vi "Transcriptor LabVIEW to C code Engine 2.vi"(7 "VI path":path, 8 "Error In":errorcluster, 11 "Diagram in":refnum<vi>) -> (0 "Error Out":errorcluster, 1 "output cluster":T1, 2 "transcripted code":string, 3 "Diagram out":refnum<vi>, 5 "VI ref.":refnum<vi>)   [LabVIEW 2014]
uses:
  types/LabVIEW Universal Transcriptor Cluster.ctl
  types/LabVIEW Universal Transcriptor C code Composer Input Cluster.ctl
panel:
  out "FiringOrder":string[](array[string])
  # "0. create definitions (ClusterConstant)\n1. get all wires and create their declarations\n2. if wires are connected to control or constant assign value to them\n3. translate elements of diagram by firing order\n4. assign values to outputs"
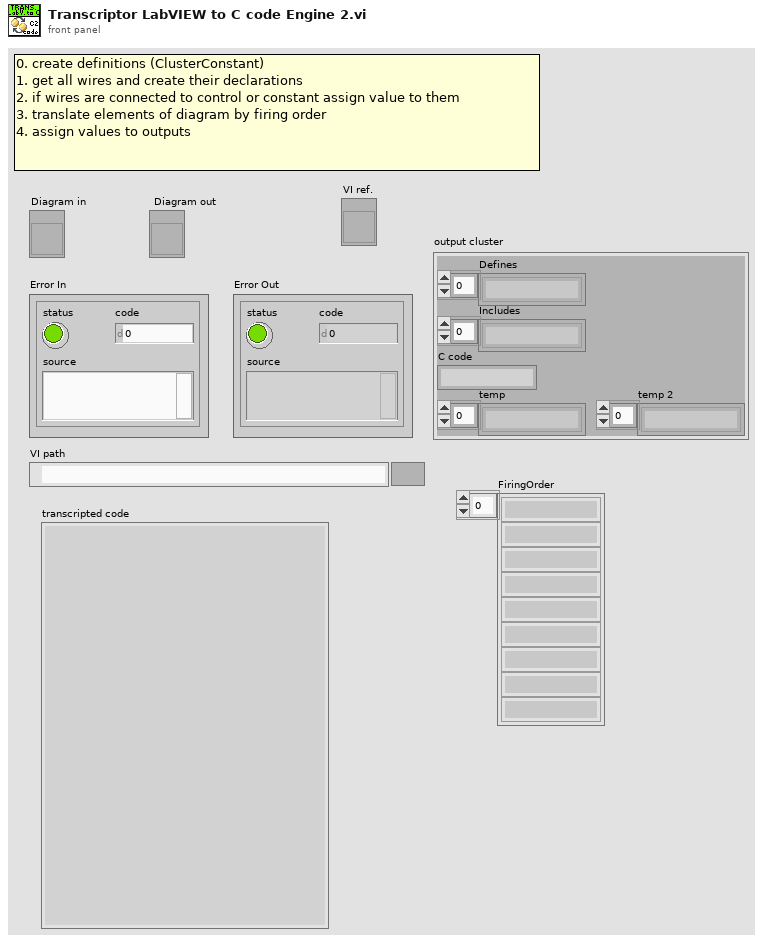
[diagram p1: front panel]
types:
  T1 = typedef "LabVIEW Universal Transcriptor Cluster.ctl" = cluster{"Defines":string[], "Includes":string[], "C code":string, "temp":string[], "temp 2":string[]}
  T2 = typedef "LabVIEW Universal Transcriptor C code Composer Input Cluster.ctl" = cluster{"structure definitions cluster":cluster{"Cluster def.":string[], "FeedbacNode def.":string[]}, "end loop refs.":string[], "wires declarations":string[], "diagram ref.":refnum<vi>, "transcriptor cluster":T1[], "feedback and other output assignments":string[], "transcripted C code":string[], "output value assignement":string}
  T3 = cluster{"Cluster def.":string[], "FeedbacNode def.":string[]}
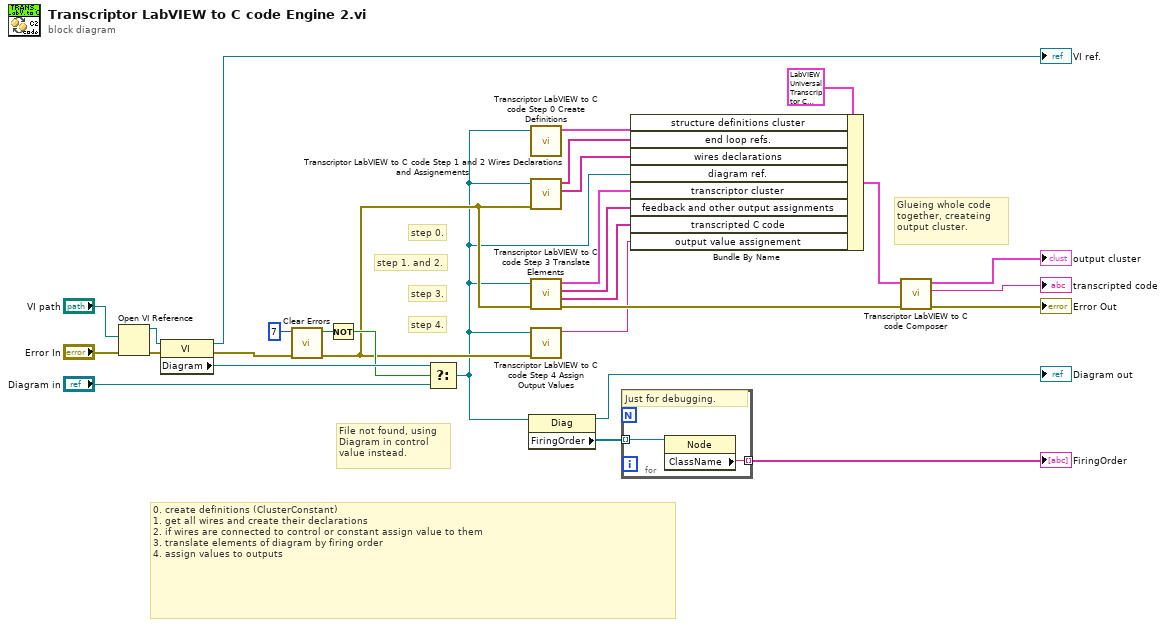
[diagram p0: block diagram]
diagram:
  # "Glueing whole code together, createing output cluster."
  # "step 4."
  # "step 3."
  # "step 1. and 2."
  # "step 0."
  # "0. create definitions (ClusterConstant)\n1. get all wires and create their declarations\n2. if wires are connected to control or constant assign value to them\n3. translate elements of diagram by firing order\n4. assign values to outputs"
  # "File not found, using Diagram in control value instead."
  n1 = Open VI Reference(vi path="VI path", error in (no error)="Error In") -> (vi reference=w18:refnum<vi>, error out=w28:errorcluster)  [unwired: 4 in]
  n2 = property on="Property Node" class="VI"(reference=w18, error in=w28) -> (reference out=→"VI ref.":refnum<vi>, error out=w25:errorcluster, "Diagram"=w27:refnum<vi>)
  n3 = call <vilib>:"Clear Errors.vi"("error in (no error)"=w25, "specific error code to clear (0: all)"=7) -> ("error out"=w20:errorcluster, "specific error cleared?"=w23:bool)  [unwired: 4 in]
  n4 = Not(x=w23) -> (.not. x?=w22:bool)
  n5 = Select(t=w27, s=w22, f="Diagram in") -> (s? t:f=w1:refnum<vi>)
  n6 = property on="Property Node" class="Diag"(reference=w1) -> (reference out=→"Diagram out":refnum<vi>, "FiringOrder"=w16:refnum<vi>[])  [unwired: 1 in, 1 out]
  n7 = call "Transcriptor LabVIEW to C code Step 0 Create Definitions.vi"("Diagram in"=w1) -> ("structure definitions cluster"=w10:T3)  [unwired: 10 in]
  n8 = call "Transcriptor LabVIEW to C code Step 1 and 2 Wires Declarations and Assignements.vi"("error in"=w20, "Diagram in"=w1) -> ("wires declarations"=w7:string[], "end loop refs."=w8:string[])  [unwired: 8 in]
  n9 = call "Transcriptor LabVIEW to C code Step 3 Translate Elements.vi"("error in (no error)"=w20, "Diagram in"=w1) -> ("error out"=w19:errorcluster, "transcripted C code"=w4:string[], "feedback and other output assignments"=w5:string[], "transcriptor cluster"=w6:T1[])  [unwired: 6 in]
  n10 = call "Transcriptor LabVIEW to C code Step 4 Assign Output Values.vi"("error in (no error)"=w20, "Diagram in"=w1) -> ("output value assignement"=w3:string)  [unwired: 9 in]
  n11 = for {
    tunnel: w16 -> [w31] mode=indexing
    tunnel: [w30] -> w26 mode=indexing
    # "Just for debugging."
    n12 = property class="Node"(reference=w31) -> ("ClassName"=w30:string)  [unwired: 1 in, 2 out]
  }
  "FiringOrder" <- w26
  n13 = Bundle By Name(cluster=T2 {"structure definitions cluster"={"Cluster def."=[], "FeedbacNode def."=[]}, "end loop refs."=[], "wires declarations"=[], "diagram ref."=refnum, "transcriptor cluster"=[], "feedback and other output assignments"=[], "transcripted C code"=[], "output value assignement"=""}, "structure definitions cluster"=w10, "end loop refs."=w8, "wires declarations"=w7, "diagram ref."=w1, "transcriptor cluster"=w6, "feedback and other output assignments"=w5, "transcripted C code"=w4, "output value assignement"=w3) -> (w11:T2)
  n14 = call "Transcriptor LabVIEW to C code Composer.vi"("error in (no error)"=w19, "C code Composer Cluster in"=w11) -> ("error out"=→"Error Out":errorcluster, "transcripted code"=→"transcripted code":string, "output cluster"=→"output cluster":T1)  [unwired: 7 in]
